vi "Button Pressed.vi"(8 "error in (no error)":errorcluster, 9 "Data":variant, 10 "Button":T1, 11 "Guardian in":refnum<class "Guardian.lvclass">) -> (0 "error out":errorcluster, 3 "Guardian out":refnum<class "Guardian.lvclass">)   [LabVIEW 2026, in "TALOS.lvlib" / "Guardian.lvlib" / "Guardian.lvclass"]
doc: "This VI execute when a message Button Pressed is invoked from the Guardian Interface (not the GUI, the Interface...)."
uses:
  Guardian.lvclass
  C:/LabVIEW Code/TALOS/builds/Actor Framework PPL/Actor Framework.lvlibp/1abvi3w/vi.lib/ActorFramework/Actor/Actor.lvclass
  C:/LabVIEW Code/TALOS/talos/Ancestor/Ancestor/Ancestor.lvclass
  Buttons_UI.ctl
  Internal uServices/System uServices/Guardian Subpanel/Launch uService Message.ctl
  Guardian Messages/Launch uService Msg/Launch uService Msg.lvclass/Launch uService Msg.ctl
  Ancestor/Ancestor/Ancestor.lvclass/Ancestor.ctl
  Classes/uService List/uService List.lvclass/uService List.ctl
  builds/Actor Framework PPL/Actor Framework.lvlibp/1abvi3w/vi.lib/ActorFramework/Message Enqueuer/Message Enqueuer.lvclass
  Guardian.lvclass/Guardian.ctl
  Guardian Messages/Message to Other Guardian Msg/Message to Other Guardian Msg.lvclass/Message to Other Guardian Msg.ctl
  Guardian Messages/TCP-SV Message Interpreter Msg/TCP-SV Message Interpreter Msg.lvclass/TCP-SV Message Interpreter Msg.ctl
  Git Update Cluster.ctl
  Guardian Messages/Message to uService Msg/Message to uService Msg.lvclass/Message to uService Msg.ctl
  Guardian Messages/Button Pressed Msg/Button Pressed Msg.lvclass/Button Pressed Msg.ctl
  Classes/uService List/Get Queue.vi
  Guardian Messages/Message to Other Guardian Msg/Send Message to Other Guardian.vi
  Ancestor/Ancestor/Read ID.vi
  Support VIs/Search Array of Strings.vi
  Guardian Messages/TCP-SV Message Interpreter Msg/Send TCP-SV Message Interpreter.vi
  Run Config Data Encoder.vi
  FGV/Error Memory/Get Error Description.vi
  Support VIs/Get PC name.vi
  Support VIs/Get Class Name.vi
  <vilib>/Utility/error.llb/Clear Errors.vi
  FGV/Error Memory/Error Memory Core.vi
  <vilib>/AdvancedString/Delimited String to 1D String Array.vi
  <vilib>/AdvancedString/Delimited String to 1D String Array (string).vi
  FGV/Error Memory/Error Crt Lvl checker.vi
  FGV/Error Memory/Error Memory Core.vi/40c8088d-b597-4017-91af-faa98e00292e.vi
  FGV/Error Memory/Error Memory Core.vi/d4a3ab98-063c-4e44-b43d-fbdcfe6c2be2.vi
  builds/Actor Framework PPL/Actor Framework.lvlibp/1abvi3w/vi.lib/ActorFramework/Message Enqueuer/Enqueue.vi
  Support VIs/Global Memory.vi
  <vilib>/Utility/LVClass/Get LV Class Name.vi
  Support VIs/Is in Packed Library.vi
  Support VIs/TALOS Root path.vi
  Support VIs/Read CSV worksheet.vi
  Support VIs/Global Constants.vi
  <vilib>/Utility/error.llb/General Error Handler.vi
  Support VIs/Error Log.vi
  Support VIs/Circus Critical PCs List.vi
  Extract uService List from CSV.vi
  Guardian Messages/Launch uService Msg/Launch uService Msg.lvclass
  Ancestor/Ancestor/Ancestor.lvclass
  <vilib>/Comparison/Equal/Equal Functor/Equal Functor.lvclass
  Guardian Messages/Message to Other Guardian Msg/Message to Other Guardian Msg.lvclass
  Guardian Messages/TCP-SV Message Interpreter Msg/TCP-SV Message Interpreter Msg.lvclass
  Guardian Messages/Message to uService Msg/Message to uService Msg.lvclass
  Guardian Messages/I Exist Msg/I Exist Msg.lvclass
  Guardian Messages/Button Pressed Msg/Button Pressed Msg.lvclass
  Classes/Guardian List/Guardian List.lvclass
  Classes/uService List/uService List.lvclass
  builds/Actor Framework PPL/Actor Framework.lvlibp/1abvi3w/vi.lib/ActorFramework/Actor/Actor.lvclass
  builds/Actor Framework PPL/Actor Framework.lvlibp/1abvi3w/vi.lib/ActorFramework/Stop Msg/Stop Msg.lvclass
  TALOS.lvlib
  Internal uServices/System uServices/Guardian Subpanel/Guardian Subpanel.lvclass
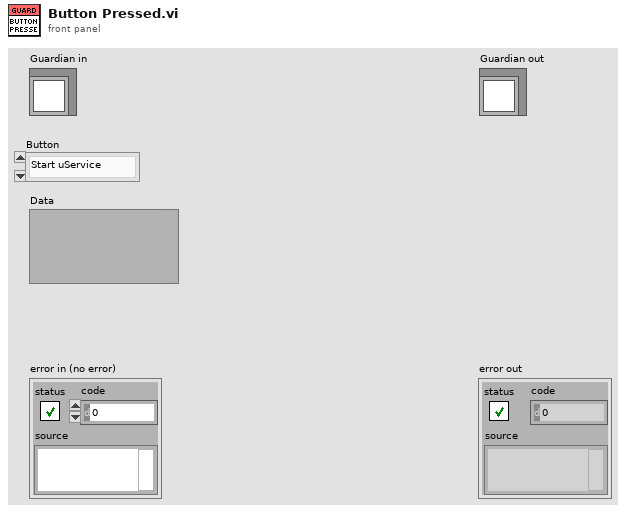
[diagram p1: front panel]
types:
  T1 = typedef "TALOS.lvlib/Guardian.lvlib/Guardian.lvclass/Buttons_UI.ctl" = enum16{"Start uService", "Kill uService", "Stop uService", "Stop", "Start online checks", "Stop online checks", "Send Pat to all GDs", "Reload INI files", "Update from GIT", "RUN", "Reset ABORT", "Check Bearer", "Send I Exist", "Change Run Config", "Add uSs from Config", "Realign uSs from Config", "Send Run Config to GD"}
  T2 = typedef "TALOS.lvlib/Guardian Subpanel.lvlib/Guardian Subpanel.lvclass/Launch uService Message.ctl" = cluster{"uService Class Name":string, "uService ID":string}
  T3 = typedef "TALOS.lvlib/Guardian.lvlib/Guardian.lvclass/Git Update Cluster.ctl" = cluster{"branch name":string, "include critical PCs":bool, "update from git":bool}
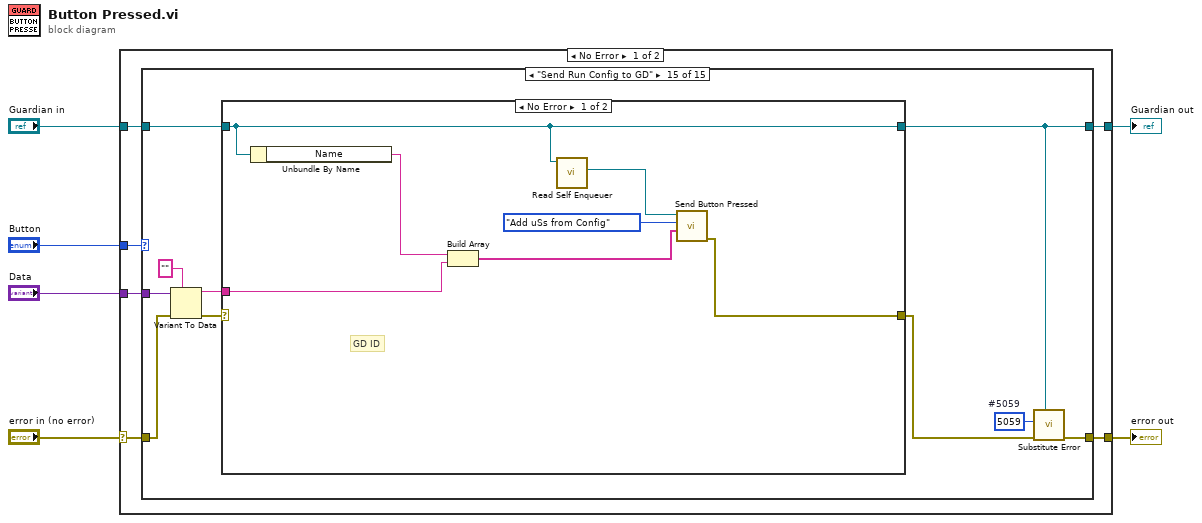
[diagram p0: block diagram]
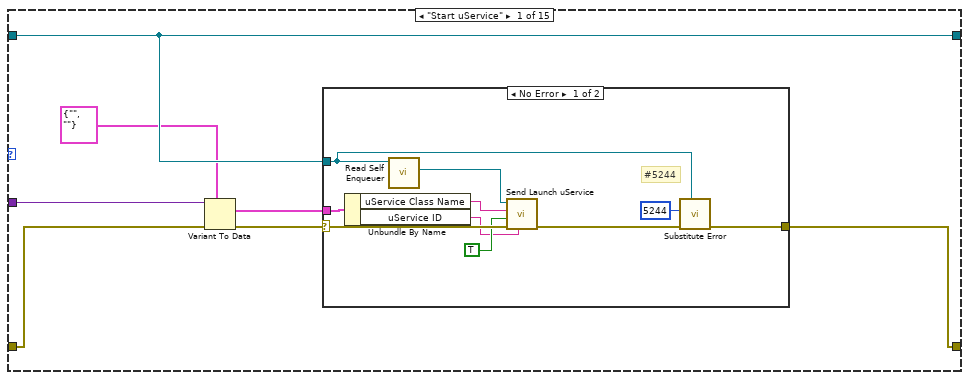
[diagram p2: hidden frame]
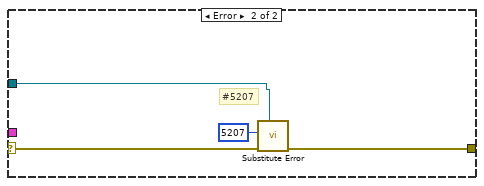
[diagram p3: hidden frame]
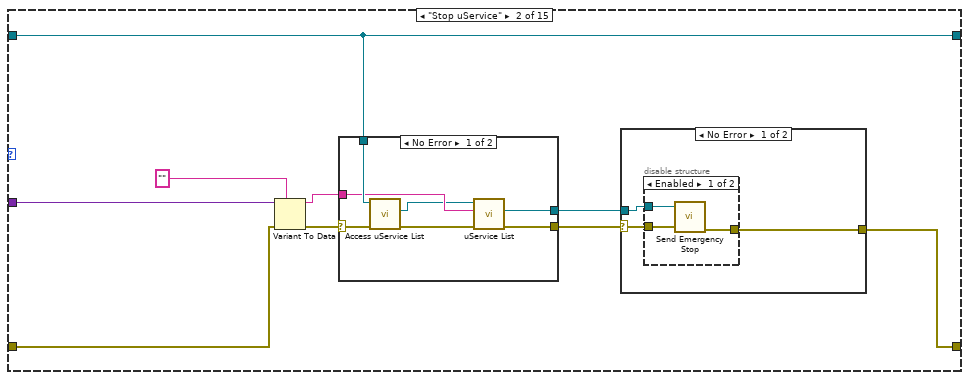
[diagram p4: hidden frame]
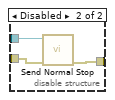
[diagram p5: hidden frame]
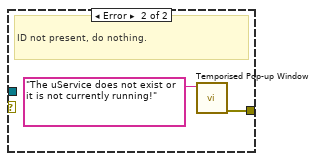
[diagram p6: hidden frame]
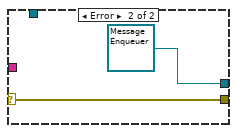
[diagram p7: hidden frame]
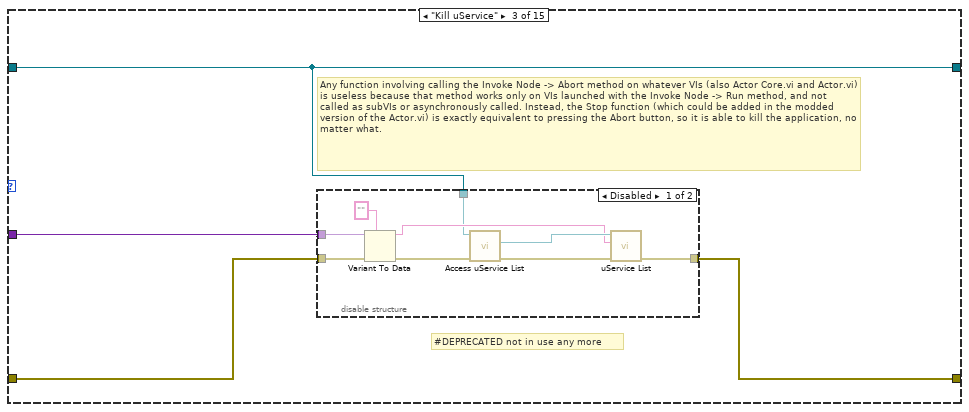
[diagram p8: hidden frame]
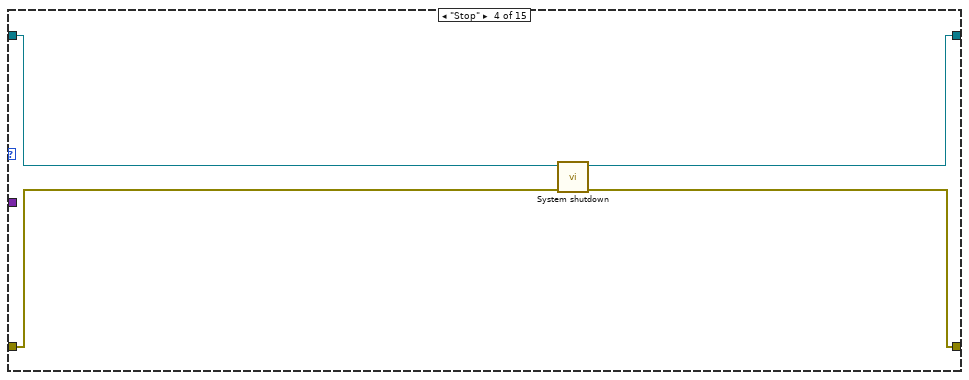
[diagram p10: hidden frame]
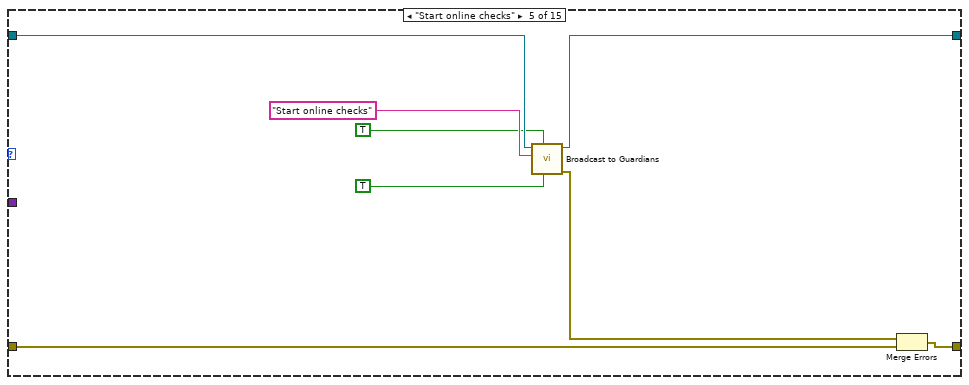
[diagram p11: hidden frame]
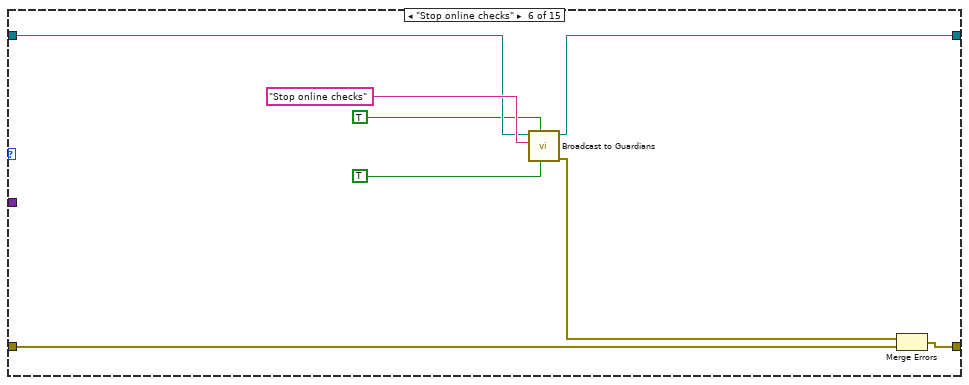
[diagram p12: hidden frame]
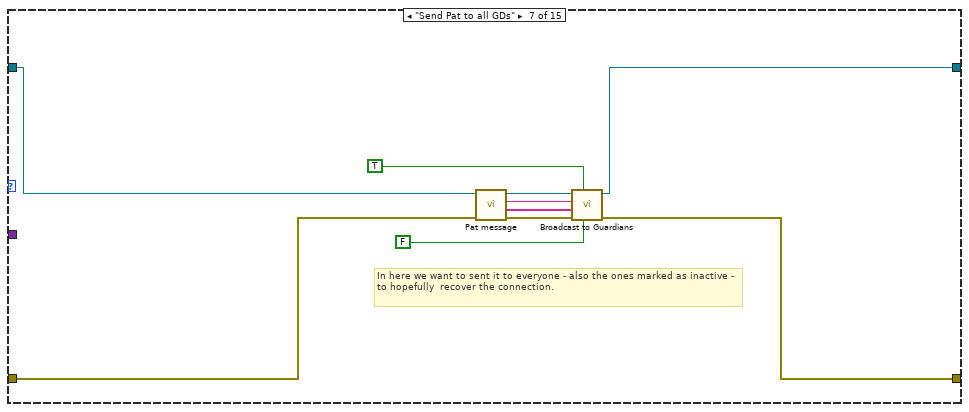
[diagram p13: hidden frame]
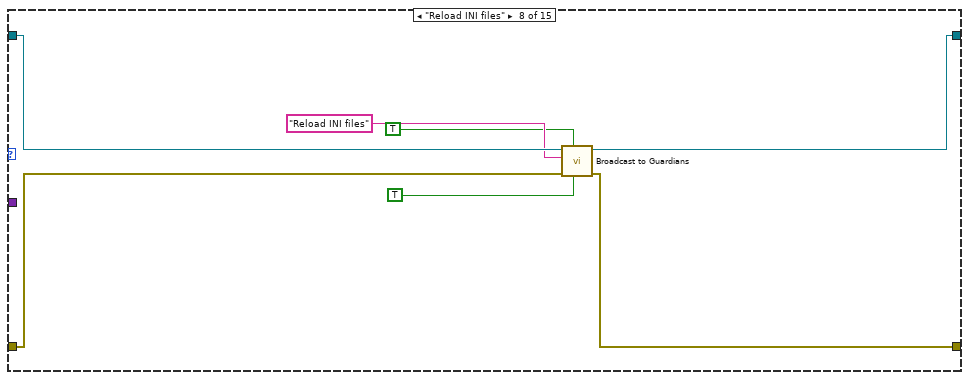
[diagram p14: hidden frame]
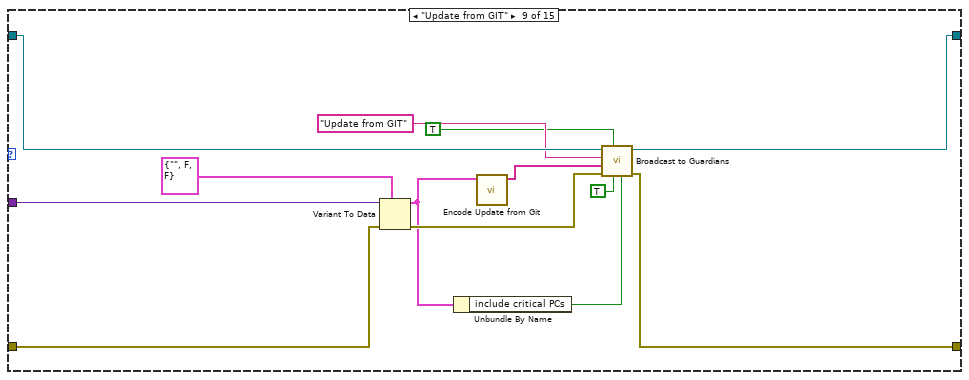
[diagram p15: hidden frame]
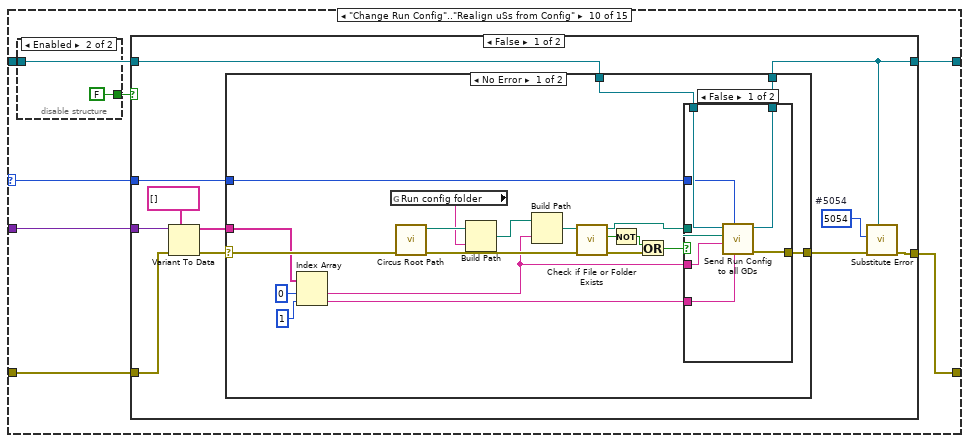
[diagram p16: hidden frame]
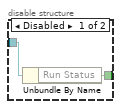
[diagram p17: hidden frame]
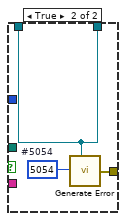
[diagram p18: hidden frame]
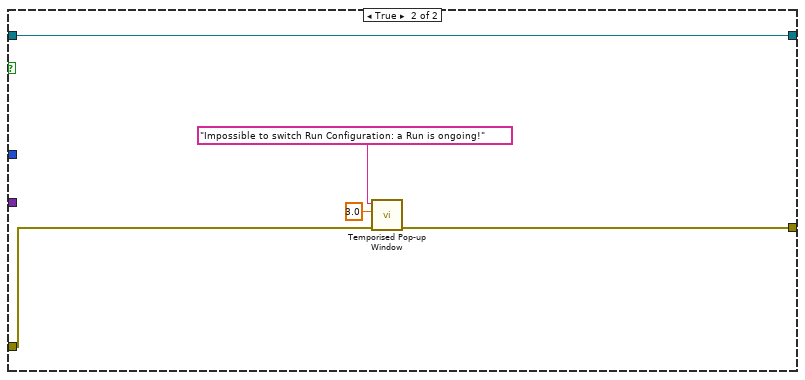
[diagram p20: hidden frame]
diagram:
  n1 = case shown="No Error" "error in (no error)" {
    selector: "error in (no error)" -> [w11 w235]
    tunnel: [w12 w235] -> w5
    tunnel: "Button" -> [w10 _]
    tunnel: [w9 w236] -> w3
    tunnel: "Guardian in" -> [w8 w236]
    tunnel: "Data" -> [w7 _]
    frame No Error {
      n2 = case shown="\"Send Run Config to GD\"" w10 {
        selector: w10 -> [_ _ _ _ _ _ _ _ _ w127 _ _ _ _ _]
        tunnel: [w14 w34 w64 w80 w86 w95 w97 w108 w124 w131 w185 w197 w198 w213 w219] -> w12
        tunnel: w11 -> [w18 w41 w65 w77 w87 w96 w99 w110 w123 w133 w186 w196 _ w210 w223]
        tunnel: [w15 w38 w63 w79 w84 w91 w98 w111 w125 w130 w187 w194 w200 w214 w216] -> w9
        tunnel: w8 -> [w15 w38 w63 w78 w88 w92 w100 w112 w126 w129 w188 w195 w200 w214 w220]
        tunnel: w7 -> [w19 w42 w66 _ _ _ _ _ w122 w132 _ _ _ _ w225]
        frame "Start uService" {
          n3 = Variant To Data(error in=w18, type=T2 {"uService Class Name"="", "uService ID"=""}, Variant=w19) -> (data=w17:T2, error out=w16:errorcluster)
          n4 = case shown="No Error" w16 {
            selector: w16 -> [w29 w32]
            tunnel: w17 -> [w22 _]
            tunnel: w15 -> [w24 w31]
            tunnel: [w23 w30] -> w14
            frame No Error {
              # "#5244"
              n5 = Unbundle By Name(w22) -> ("uService Class Name"=w21:string, "uService ID"=w20:string)
              n6 = call "Read Self Enqueuer.vi"("Actor"=w24) -> ("Self Enqueuer"=w28:refnum<class "Message Enqueuer.lvclass">)  [unwired: 10 in]
              n7 = call "Send Launch uService.vi"("uService ID"=w20, "error in (no error)"=w29, "GUI?"=TRUE, "uService Class Name"=w21, "Message Enqueuer"=w28) -> ("error out"=w25:errorcluster)  [unwired: 5 in, 1 out]
              n8 = call "Substitute Error.vi"("LabVIEW Object"=w24, "error in (no error)"=w25, "Error Code"=5244) -> ("error out"=w23:errorcluster)  [unwired: 8 in]
            }
            frame Error {
              # "#5207"
              n9 = call "Substitute Error.vi"("LabVIEW Object"=w31, "error in (no error)"=w32, "Error Code"=5207) -> ("error out"=w30:errorcluster)  [unwired: 8 in]
            }
          }
        }
        frame "Stop uService" {
          n10 = Variant To Data(error in=w41, type="", Variant=w42) -> (data=w37:string, error out=w39:errorcluster)
          n11 = case shown="No Error" w39 {
            selector: w39 -> [w60 w62]
            tunnel: w38 -> [w58 _]
            tunnel: w37 -> [w57 _]
            tunnel: [w55 w62] -> w36
            tunnel: [w54 refnum<class "Message Enqueuer.lvclass"> refnum ("uService Queue")] -> w35
            frame No Error {
              n12 = call-dynamic "Access uService List.vi"("error in (no error)"=w60, "Ancestor in"=w58) -> ("error out"=w59:errorcluster, "uService List out"=w56:refnum<class "uService List.lvclass">)  [unwired: 7 in, 1 out]
              n13 = call-poly "uService List.vi"("error in (no error)"=w59, "ID"=w57, "uService List in"=w56) -> ("error out"=w55:errorcluster, "uService Queue"=w54:refnum<class "Message Enqueuer.lvclass">)  [unwired: 6 in, 1 out]
            }
            frame Error {
            }
          }
          n14 = case shown="No Error" w36 {
            selector: w36 -> [w43 _]
            tunnel: w35 -> [w45 _]
            tunnel: [w44 w53] -> w34
            frame No Error {
              n15 = disable-structure shown="Enabled" {
                disable-tunnel: w43 -> [w48 w51]
                disable-tunnel: w45 -> [w46 w49]
                disable-tunnel: [w47 w50] -> w44
                frame Enabled {
                  n16 = call "Send Emergency Stop.vi"("error in (no error)"=w48, "Message Enqueuer"=w46) -> ("error out"=w47:errorcluster)  [unwired: 9 in]
                }
                frame Disabled {
                  n17 = call "Send Normal Stop.vi"("error in (no error)"=w51, "Message Enqueuer"=w49) -> ("error out"=w50:errorcluster)  [unwired: 9 in]
                }
              }
            }
            frame Error {
              # "ID not present, do nothing."
              n18 = call "Temporised Pop-up Window.vi"("Text"="The uService does not exist or it is not currently running!") -> ("error out"=w53:errorcluster)  [unwired: 10 in]
            }
          }
        }
        frame "Kill uService" {
          # "#DEPRECATED not in use any more"
          # "Any function involving calling the Invoke Node -> Abort method on whatever VIs (also Actor Core.vi and Actor.vi) is useless because that method works only on VIs launched with the Invoke Node -> Run method, and not called as subVIs or asynchronously called. Instead, the Stop function (which could be added in the modded version of the Actor.vi) is exactly equivalent to pressing the Abort button, so it is able to kill the application, no matter what."
          n19 = disable-structure shown="Disabled" {
            disable-tunnel: w66 -> [w74 _]
            disable-tunnel: w65 -> [w73 w76]
            disable-tunnel: [w72 w76] -> w64
            disable-tunnel: w63 -> [w67 _]
            frame Disabled {
              n20 = Variant To Data(error in=w73, type="", Variant=w74) -> (data=w68:string, error out=w71:errorcluster)
              n21 = call-dynamic "Access uService List.vi"("error in (no error)"=w71, "Ancestor in"=w67) -> ("error out"=w70:errorcluster, "uService List out"=w69:refnum<class "uService List.lvclass">)  [unwired: 7 in, 1 out]
              n22 = call-poly "uService List.vi"("error in (no error)"=w70, "ID"=w68, "uService List in"=w69) -> ("error out"=w72:errorcluster)  [unwired: 6 in, 2 out]
            }
            frame Enabled {
            }
          }
        }
        frame "Stop" {
          n23 = call "System shutdown.vi"("error in (no error)"=w77, "Guardian in"=w78) -> ("error out"=w80:errorcluster, "Guardian out"=w79:refnum<class "Guardian.lvclass">)  [unwired: 8 in]
        }
        frame "Start online checks" {
          n24 = call "Broadcast to Guardians.vi"("Only active ones?"=TRUE, "Local also?"=TRUE, "Message"="Start online checks", "Guardian in"=w88) -> ("error out"=w83:errorcluster, "Guardian out"=w84:refnum<class "Guardian.lvclass">)  [unwired: 6 in]
          n25 = Merge Errors(w83, w87) -> (w86:errorcluster)
        }
        frame "Stop online checks" {
          n26 = call "Broadcast to Guardians.vi"("Only active ones?"=TRUE, "Local also?"=TRUE, "Message"="Stop online checks", "Guardian in"=w92) -> ("error out"=w93:errorcluster, "Guardian out"=w91:refnum<class "Guardian.lvclass">)  [unwired: 6 in]
          n27 = Merge Errors(w93, w96) -> (w95:errorcluster)
        }
        frame "Send Pat to all GDs" {
          # "In here we want to sent it to everyone - also the ones marked as inactive - to hopefully  recover the connection."
          n28 = call "Pat message.vi"("error in (no error)"=w99, "Guardian in"=w100) -> ("error out"=w105:errorcluster, "Data"=w104:string[], "Message name"=w102:string, "Guardian out"=w106:refnum<class "Guardian.lvclass">)  [unwired: 6 in]
          n29 = call "Broadcast to Guardians.vi"("Only active ones?"=FALSE, "Local also?"=TRUE, "error in (no error)"=w105, "Data"=w104, "Message"=w102, "Guardian in"=w106) -> ("error out"=w97:errorcluster, "Guardian out"=w98:refnum<class "Guardian.lvclass">)  [unwired: 4 in]
        }
        frame "Reload INI files" {
          n30 = call "Broadcast to Guardians.vi"("Only active ones?"=TRUE, "Local also?"=TRUE, "error in (no error)"=w110, "Message"="Reload INI files", "Guardian in"=w112) -> ("error out"=w108:errorcluster, "Guardian out"=w111:refnum<class "Guardian.lvclass">)  [unwired: 5 in]
        }
        frame "Update from GIT" {
          n31 = Variant To Data(error in=w123, type=T3 {"branch name"="", "include critical PCs"=FALSE, "update from git"=FALSE} ("Git update cluster"), Variant=w122) -> (data=w115:T3, error out=w121:errorcluster)
          n32 = Unbundle By Name(w115) -> ("include critical PCs"=w116:bool)
          n33 = call "Encode Update from Git.vi"("Git update cluster"=w115) -> ("Encoded message"=w114:string[])  [unwired: 10 in]
          n34 = call "Broadcast to Guardians.vi"("Critical PCs also?"=w116, "Only active ones?"=TRUE, "Local also?"=TRUE, "error in (no error)"=w121, "Data"=w114, "Message"="Update from GIT", "Guardian in"=w126) -> ("error out"=w124:errorcluster, "Guardian out"=w125:refnum<class "Guardian.lvclass">)  [unwired: 3 in]
        }
        frame "Change Run Config".."Realign uSs from Config" {
          n35 = disable-structure shown="Enabled" {
            disable-tunnel: w129 -> [w135 _]
            disable-tunnel: [w134 FALSE ("Run Status")] -> w128
            frame Disabled {
              n36 = Unbundle By Name(w135) -> ("Run Status"=w134:bool)
            }
            frame Enabled {
            }
          }
          n37 = case shown="False" w128 {
            tunnel: w129 -> [w147 w180]
            tunnel: w133 -> [w146 w184]
            tunnel: w132 -> [w145 _]
            tunnel: [w140 w183] -> w131
            tunnel: [w139 w180] -> w130
            tunnel: w127 -> [w137 _]
            frame False {
              w138 = 5054  # #5054
              n38 = Variant To Data(error in=w146, type=string[] [], Variant=w145) -> (data=w142:string[], error out=w143:errorcluster)
              n39 = case shown="No Error" w143 {
                selector: w143 -> [w162 w179]
                tunnel: w147 -> [w167 w178]
                tunnel: [w166 w178] -> w139
                tunnel: [w155 w179] -> w141
                tunnel: w142 -> [w154 _]
                tunnel: w137 -> [w153 _]
                frame No Error {
                  n40 = Index Array(array=w154, index #1=0 ("index"), index #2=1 ("index")) -> (element #1=w151:string, element #2=w148:string)
                  n41 = global read "Global Constants.vi" "Run config folder"() -> (w163:string)
                  n42 = call "Circus Root Path.vi"("error in (no error)"=w162) -> ("error out"=w160:errorcluster, "Circus Root Path"=w164:path)  [unwired: 9 in]
                  n43 = Build Path(base path=w164, name or relative path=w163) -> (appended path=w165:path)
                  n44 = Build Path(base path=w165, name or relative path=w151) -> (appended path=w161:path)
                  n45 = call <vilib>:"Check if File or Folder Exists.vi"("error in (no error)"=w160, "path"=w161) -> ("error out"=w159:errorcluster, "file or folder exists?"=w158:bool, "dup path"=w152:path)  [unwired: 7 in]
                  n46 = Not(x=w158) -> (.not. x?=w157:bool)
                  n47 = Or(x=w157, y=w159) -> (x .or. y?=w156:bool)
                  n48 = case shown="False" w156 {
                    tunnel: w167 -> [w174 w177]
                    tunnel: [w173 w177] -> w166
                    tunnel: [w172 w176] -> w155
                    tunnel: w151 -> [w169 _]
                    tunnel: w153 -> [w171 _]
                    tunnel: w152 -> [w170 _]
                    tunnel: w148 -> [w168 _]
                    frame False {
                      n49 = call "Send Run Config to all GDs.vi"("Guardian ID or ALL"=w168, "Button"=w171, "Run Config Name"=w169, "CSV Path"=w170, "Guardian in"=w174) -> ("error out"=w172:errorcluster, "Guardian out"=w173:refnum<class "Guardian.lvclass">)  [unwired: 5 in]
                    }
                    frame True {
                      w175 = 5054  # #5054
                      n50 = call "Generate Error.vi"("Class"=w177, "Error Code"=w175) -> ("error out"=w176:errorcluster)  [unwired: 5 in]
                    }
                  }
                }
                frame Error {
                }
              }
              n51 = call "Substitute Error.vi"("LabVIEW Object"=w139, "error in (no error)"=w141, "Error Code"=w138) -> ("error out"=w140:errorcluster)  [unwired: 8 in]
            }
            frame True {
              n52 = call "Temporised Pop-up Window.vi"("error in (no error)"=w184, "Timeout"=3.0, "Text"="Impossible to switch Run Configuration: a Run is ongoing!") -> ("error out"=w183:errorcluster)  [unwired: 8 in]
            }
          }
        }
        frame "RUN" {
          n53 = call "Broadcast to Guardians.vi"("Only active ones?"=TRUE, "Local also?"=TRUE, "error in (no error)"=w186, "Message"="Reset Run LED", "Guardian in"=w188) -> ("error out"=w185:errorcluster, "Guardian out"=w187:refnum<class "Guardian.lvclass">)  [unwired: 5 in]
        }
        frame "Reset ABORT" {
          n54 = call "Raise or Lower Abort.vi"("error in (no error)"=w196, "Sender"="local", "New Abort Value"=FALSE, "Guardian in"=w195) -> ("error out"=w197:errorcluster, "Guardian out"=w194:refnum<class "Guardian.lvclass">)  [unwired: 6 in]
        }
        frame "Check Bearer" {
          # "#5244"
          n55 = Unbundle By Name(w200) -> ("GD Subpanel ID"=w207:string, "Bearer"=w205:string)
          n56 = call "Read Self Enqueuer.vi"("Actor"=w200) -> ("Self Enqueuer"=w209:refnum<class "Message Enqueuer.lvclass">)  [unwired: 10 in]
          n57 = call "Date n Time.vi"() -> ("Date & Time"=w203:string)  [unwired: 5 in]
          n58 = call <vilib>:"Space Constant.vi"() -> ("String"=w204:string)
          n59 = Concatenate Strings(w205, w204, w203) -> (w202:string)
          n60 = call "Send Message to uService.vi"("uService ID"=w207, "Message"="Update Bearer", "Data"=w202, "Locale?"=TRUE, "Message Enqueuer"=w209) -> ("error out"=w199:errorcluster)  [unwired: 5 in, 1 out]
          n61 = call "Substitute Error.vi"("LabVIEW Object"=w200, "error in (no error)"=w199, "Error Code"=5244) -> ("error out"=w198:errorcluster)  [unwired: 8 in]
        }
        frame "Send I Exist" {
          # "#5244"
          n62 = call "Read Self Enqueuer.vi"("Actor"=w214) -> ("Self Enqueuer"=w212:refnum<class "Message Enqueuer.lvclass">)  [unwired: 10 in]
          n63 = call "Send I Exist.vi"("error in (no error)"=w210, "Message Enqueuer"=w212) -> ("error out"=w211:errorcluster)  [unwired: 8 in, 1 out]
          n64 = call "Substitute Error.vi"("LabVIEW Object"=w214, "error in (no error)"=w211, "Error Code"=5244) -> ("error out"=w213:errorcluster)  [unwired: 8 in]
        }
        frame "Send Run Config to GD" {
          w218 = 5059  # #5059
          n65 = Variant To Data(error in=w223, type="", Variant=w225) -> (data=w221:string, error out=w224:errorcluster)
          n66 = case shown="No Error" w224 {
            selector: w224 -> [_ w233]
            tunnel: w221 -> [w231 _]
            tunnel: w220 -> [w227 w234]
            tunnel: [w227 w234] -> w216
            tunnel: [w228 w233] -> w217
            frame No Error {
              # "GD ID"
              n67 = Unbundle By Name(w227) -> ("Name"=w232:string)
              n68 = Build Array(w232, w231) -> (w229:string[])
              n69 = call "Read Self Enqueuer.vi"("Actor"=w227) -> ("Self Enqueuer"=w226:refnum<class "Message Enqueuer.lvclass">)  [unwired: 10 in]
              n70 = call "Send Button Pressed.vi"("Data"=w229, "Button"=Buttons_UI."Add uSs from Config", "Message Enqueuer"=w226) -> ("error out"=w228:errorcluster)  [unwired: 7 in, 1 out]
            }
            frame Error {
            }
          }
          n71 = call "Substitute Error.vi"("LabVIEW Object"=w216, "error in (no error)"=w217, "Error Code"=w218) -> ("error out"=w219:errorcluster)  [unwired: 8 in]
        }
      }
    }
    frame Error {
    }
  }
  "error out" <- w5
  "Guardian out" <- w3
